vi "Unsubscribe (async).vi"(8 "error in (no error)":errorcluster, 9 "Topic":string, 11 "WAMP Client in":refnum<class "WAMP Client.lvclass">) -> (0 "error out":errorcluster, 1 "Result Event":refnum<user-event>, 3 "WAMP Client out":refnum<class "WAMP Client.lvclass">)   [LabVIEW 2020, in "wamplv.lvlib" / "WAMP Client.lvclass"]
uses:
  WAMP Client.lvclass
  WAMP Client.lvclass/WAMP Client.ctl
  TypeDef/UNSUBSCRIBE Result.ctl
  TypeDef/UNSUBSCRIBE Request Data.ctl
  TypeDef/Internal Message Type.ctl
  API/TypeDefs/WAMP error.ctl
  API/TypeDefs/Combined error.ctl
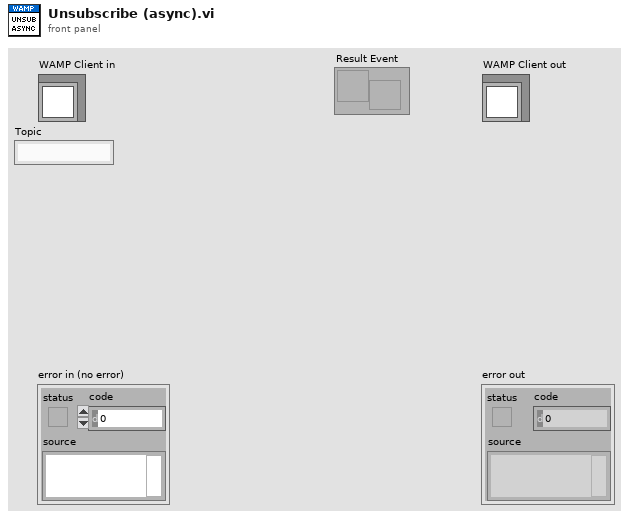
[diagram p1: front panel]
types:
  T1 = typedef "wamplv.lvlib/WAMP Client.lvclass/Internal Message Type.ctl" = enum16{"Subscribe", "Handle Subscribed", "Handle Event", "Unsubscribe", "Handle Unsubscribed", "Publish", "Handled Published", "Goodbye", "Handle Goodbye", "Call", "Handle Result", "Register", "Handle Registered", "Unregister", "Handle Unregistered", "Handle Invocation", "Yield", "Error"}
  T2 = typedef "wamplv.lvlib/WAMP Client.lvclass/UNSUBSCRIBE Request Data.ctl" = cluster{"Topic":string, "Unsubscribe Result Received Event":refnum<user-event>}
  T3 = typedef "wamplv.lvlib/WAMP Client.lvclass/UNSUBSCRIBE Result.ctl" = cluster{"Success?":bool, "Combined Error":T4}
  T4 = typedef "wamplv.lvlib/WAMP Client.lvclass/Combined error.ctl" = cluster{"Error?":bool, "WAMP Error":T5, "Error":errorcluster}
  T5 = typedef "wamplv.lvlib/WAMP Client.lvclass/WAMP error.ctl" = cluster{"Details":string, "ArgumentKw Payload":string, "Error?":bool, "Error URI":string, "Arguments Payload":string[]}
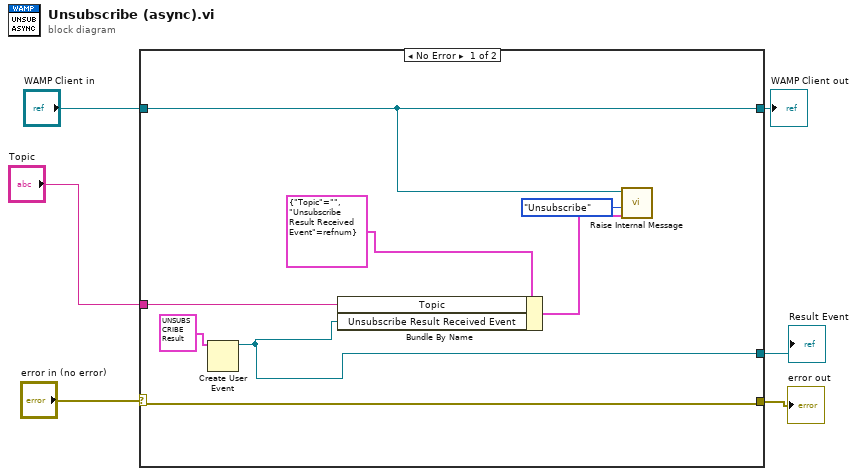
[diagram p0: block diagram]
diagram:
  n1 = case shown="No Error" "error in (no error)" {
    selector: "error in (no error)" -> [w14 w16]
    tunnel: [w14 w16] -> w5
    tunnel: [w13 w15] -> w3
    tunnel: "WAMP Client in" -> [w13 w15]
    tunnel: [w8 _] -> w1
    tunnel: "Topic" -> [w11 _]
    frame No Error {
      n2 = Create User Event(user event datatype=T3 {"Success?"=FALSE, "Combined Error"={"Error?"=FALSE, "WAMP Error"={"Details"="", "ArgumentKw Payload"="{}", "Error?"=FALSE, "Error URI"="", "Arguments Payload"=[]}, "Error"={"status"=FALSE, "code"=0, "source"=""}}} ("Subcsribe Result")) -> (user event=w8:refnum<user-event>)  [unwired: 1 in, 1 out]
      n3 = Bundle By Name(cluster=T2 {"Topic"="", "Unsubscribe Result Received Event"=refnum} ("Cluster"), "Topic"=w11, "Unsubscribe Result Received Event"=w8) -> (w12:T2)
      n4 = call-dynamic "Raise Internal Message.vi"("Variant"=w12, "Internal Message Type"=Internal_Message_Type."Unsubscribe", "WAMP Client in"=w13) -> ()  [unwired: 7 in, 2 out]
    }
    frame Error {
    }
  }
  "error out" <- w5
  "WAMP Client out" <- w3
  "Result Event" <- w1
